vi "Set Cell View.vi"(8 "error in (no error)":errorcluster, 10 "Cell View":refnum<k24>, 11 "Cell View in":refnum<class "Cell View.lvclass">) -> (0 "error out":errorcluster, 3 "Cell View out":refnum<class "Cell View.lvclass">)   [LabVIEW 2024, in "Cell View.lvclass"]
uses:
  Cell View.lvclass
  D:/git/Sourcegrid-LabVIEW/dll/SourceGrid.dll
  dll/SourceGrid.dll
  Cell View.lvclass/Cell View.ctl
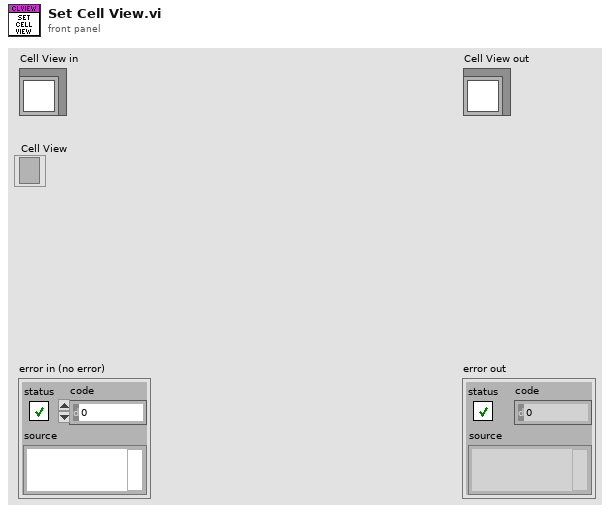
[diagram p1: front panel]
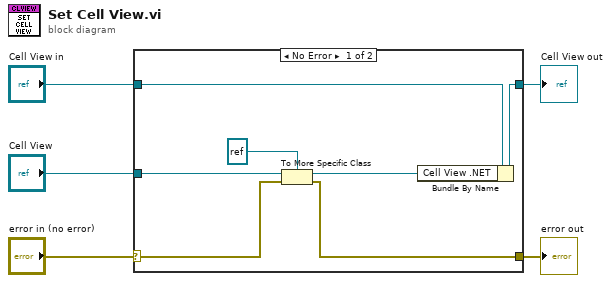
[diagram p0: block diagram]
diagram:
  n1 = case shown="No Error" "error in (no error)" {
    selector: "error in (no error)" -> [w8 w13]
    tunnel: [w7 w13] -> w4
    tunnel: [w11 w14] -> w2
    tunnel: "Cell View in" -> [w12 w14]
    tunnel: "Cell View" -> [w10 _]
    frame No Error {
      n2 = To More Specific Class(target class=refnum<k24> refnum ("new reference"), reference=w10, error in=w8) -> (specific class reference=w9:refnum<k24>, error out=w7:errorcluster)
      n3 = Bundle By Name(cluster=w12, "Cell View .NET"=w9) -> (w11:refnum<class "Cell View.lvclass">)
    }
    frame Error {
    }
  }
  "error out" <- w4
  "Cell View out" <- w2
